vi "15-DP.vi"() -> ()   [LabVIEW 2021]
panel:
  out "Number of Lattice Paths":u64
  in  "Number of Columns":i32=20
  in  "Number of Rows":i32=20
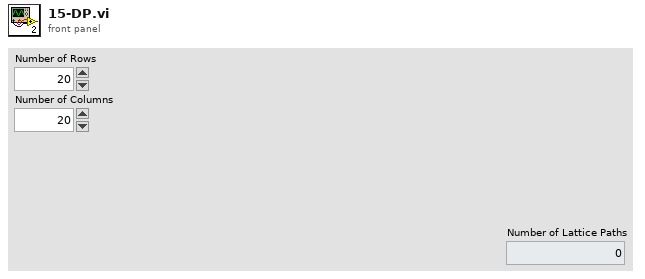
[diagram p1: front panel]
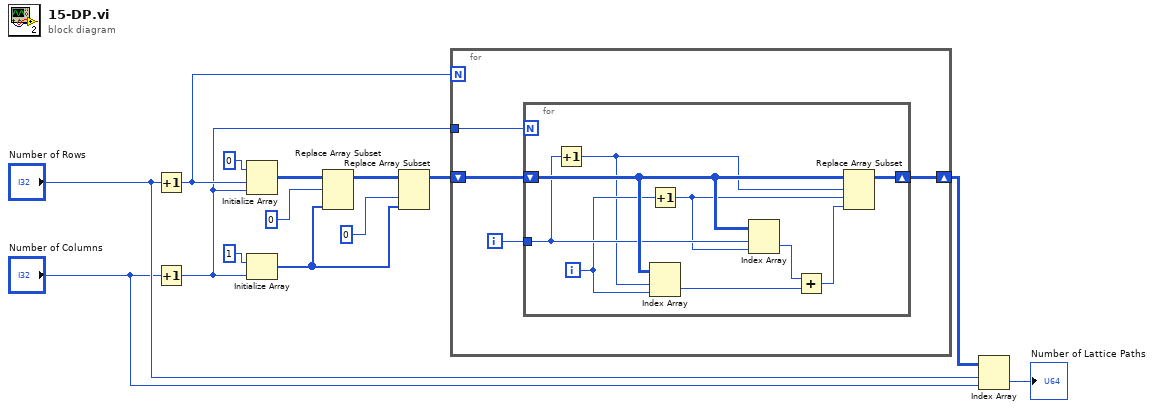
[diagram p0: block diagram]
diagram:
  n1 = Increment(x="Number of Rows") -> (x+1=w5:i32)
  n2 = Increment(x="Number of Columns") -> (x+1=w4:i32)
  n3 = Initialize Array(u64 0, w5, w4) -> (w8:u64[][])
  n4 = Initialize Array(u64 1, w4) -> (w10:u64[])
  n5 = Replace Array Subset(array=w8, new element=w10, index (row)=0) -> (w9:u64[][])  [unwired: 1 in]
  n6 = Replace Array Subset(array=w9, new element=w10, index (col)=0) -> (w7:u64[][])  [unwired: 1 in]
  n7 = for {
    N: w5 -> [_]
    tunnel: w4 -> [w17]
    shift-right: [w16] -> w6
    shift-left: w7 -> [w18]
    i -> [w15]
    n8 = for {
      N: w17 -> [_]
      shift-right: [w27] -> w16
      shift-left: w18 -> [w26]
      tunnel: w15 -> [w25]
      i -> [w24]
      n9 = Increment(x=w25) -> (x+1=w19:i32)
      n10 = Increment(x=w24) -> (x+1=w20:i32)
      n11 = Index Array(array=w26, index (row)=w19, index (col)=w24) -> (element=w22:u64)
      n12 = Index Array(array=w26, index (row)=w25, index (col)=w20) -> (element=w23:u64)
      n13 = Add(x=w23, y=w22) -> (x+y=w21:u64)
      n14 = Replace Array Subset(array=w26, new element=w21, index (row)=w19, index (col)=w20) -> (w27:u64[][])
    }
  }
  n15 = Index Array(array=w6, index (row)="Number of Rows", index (col)="Number of Columns") -> (element=→"Number of Lattice Paths":u64)
